vi "Intake Get and use.vi"(2 "TakeBall":dbl, 3 "Cannon vbus":dbl, 4 "Upper Claw":dbl) -> (0 "Intake Info Out":T1, 1 "InTake Max":bool)   [LabVIEW 2013]
uses:
  Intake Global.vi
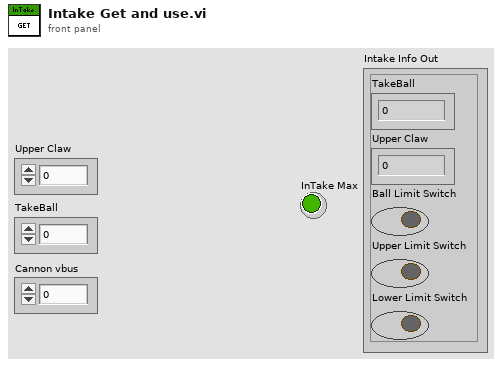
[diagram p1: front panel]
types:
  T1 = cluster{"TakeBall":dbl, "Upper Claw":dbl, "Ball Limit Switch":bool, "Upper Limit Switch":bool, "Lower Limit Switch ":bool}
  T2 = cluster{"TakeBall":dbl, "Upper Claw":dbl, "Ball In Cannon?":bool, "InTake Max":bool, "InTake Min":bool}
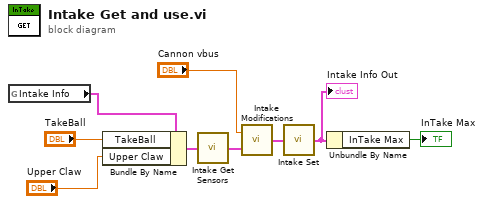
[diagram p0: block diagram]
diagram:
  n1 = global read "Intake Global.vi" "Intake Info"() -> (w9:T2)
  n2 = Bundle By Name(cluster=w9, "TakeBall"="TakeBall", "Upper Claw"="Upper Claw") -> (w6:T2)
  n3 = call "Intake Get Sensors.vi"("Intake Info In"=w6) -> ("Intake Info In"=w5:T2)
  n4 = call "Intake Modifications.vi"("Intake Info In"=w5, "Cannon vbus"="Cannon vbus") -> ("Intake Info In"=w2:T2)
  n5 = call "Intake Set.vi"("Intake Info In"=w2) -> ("Intake Info In"=w1:T2)
  "Intake Info Out" <- w1
  n6 = Unbundle By Name(w1) -> ("InTake Max"=→"InTake Max":bool)
